vi "SFTP File Type.vi"(1 "permissions":u32) -> (0 "type":T1)   [LabVIEW 2017, in "libssh2.lvlib"]
doc: "Returns the type of a file from the specified permissions."
uses:
  libssh2.lvlib
  SFTP File Type.ctl
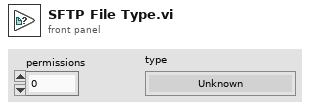
[diagram p1: front panel]
types:
  T1 = typedef "libssh2.lvlib/SFTP File Type.ctl" = enum16{"Unknown", "Named Pipe (FIFO)", "Character Special File", "Directory", "Block Special File", "Regular File", "Symbolic Link", "Socket"}
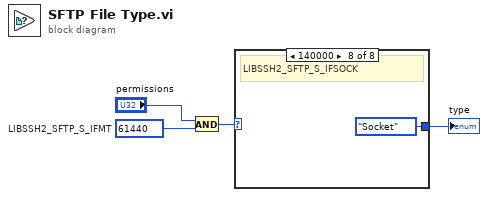
[diagram p0: block diagram]
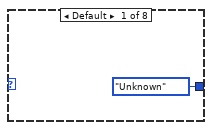
[diagram p2: hidden frame]
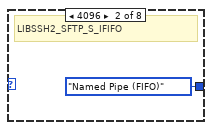
[diagram p3: hidden frame]
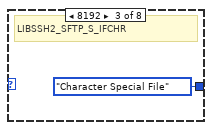
[diagram p4: hidden frame]
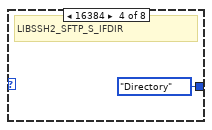
[diagram p5: hidden frame]
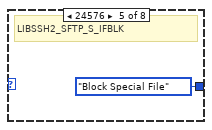
[diagram p6: hidden frame]
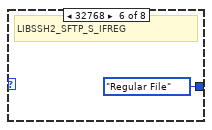
[diagram p7: hidden frame]
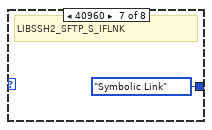
[diagram p8: hidden frame]
diagram:
  w4 = u32 61440  # LIBSSH2_SFTP_S_IFMT
  n1 = And(x="permissions", y=w4) -> (x .and. y?=w3:u32)
  n2 = case shown="140000" w3 {
    tunnel: [SFTP_File_Type."Unknown" ("type") SFTP_File_Type."Named Pipe (FIFO)" ("type") SFTP_File_Type."Character Special File" ("type") SFTP_File_Type."Directory" ("type") SFTP_File_Type."Block Special File" ("type") SFTP_File_Type."Regular File" ("type") SFTP_File_Type."Symbolic Link" ("type") SFTP_File_Type."Socket" ("type")] -> w2
    frame Default {
    }
    frame 4096 {
      # "LIBSSH2_SFTP_S_IFIFO"
    }
    frame 8192 {
      # "LIBSSH2_SFTP_S_IFCHR"
    }
    frame 16384 {
      # "LIBSSH2_SFTP_S_IFDIR"
    }
    frame 24576 {
      # "LIBSSH2_SFTP_S_IFBLK"
    }
    frame 32768 {
      # "LIBSSH2_SFTP_S_IFREG"
    }
    frame 40960 {
      # "LIBSSH2_SFTP_S_IFLNK"
    }
    frame 49152 {
      # "LIBSSH2_SFTP_S_IFSOCK"
    }
  }
  "type" <- w2
